vi "Traverse_to_Traverse_Collision.vi"(5 "Current Position":sgl[](array[numeric])=[0.0, 100.0, 40.0] format="%.2f", 7 "Traverse Name":string, 8 "Model  Roll        Pitch       Yaw (deg)":sgl[](array[numeric]) format="%#.2f", 9 "Work in Tunnel Coordinates":T1, 10 "Simulate/Run":T2=enum."Run VI", 11 "New Position":sgl[](array[numeric])=[0.0, 100.0, 40.0] format="%.2f") -> (1 "Error String":string)   [LabVIEW 2015]
uses:
  Controls/User_Specific_mode.ctl
  Controls/Tunnel_Coordinates.ctl
  Route mapping/Exclude_cluster.ctl
  Route mapping/Box_size.ctl
  Route mapping/Exclusion_type.ctl
  ADAM Client/Sub VIs/ADAM Controls/Quick_local_ADAM_Table.ctl
  Route mapping/Pict_Plot_Axis.ctl
  Route mapping/Axis.ctl
  Globals/Preference_global.vi
  Globals/Trav_pos_global.vi
panel:
  out "Plan View":picture
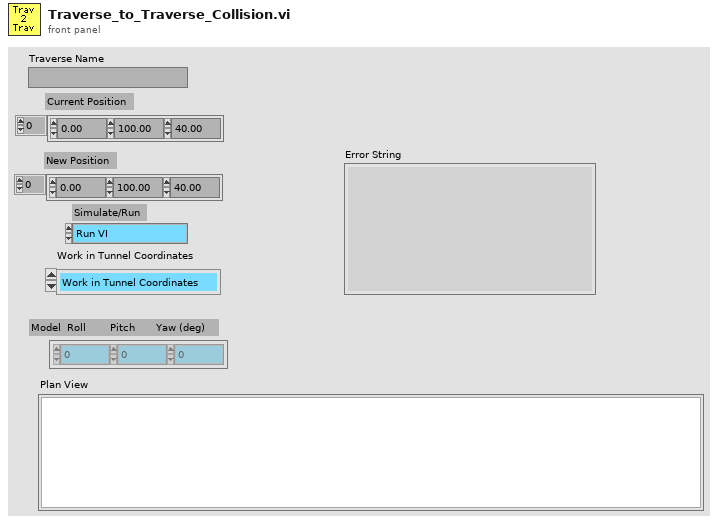
[diagram p1: front panel]
types:
  T1 = typedef "Tunnel_Coordinates.ctl" = enum16{"Work in Tunnel Coordinates", "Work in Model Coordinates"}
  T2 = typedef "User_Specific_mode.ctl" = enum16{"Check VI only", "Run VI"}
  T3 = typedef "Exclude_cluster.ctl" = cluster{"Sizes":T4, "Name":string, "Exclude Type":T5}
  T4 = typedef "Box_size.ctl" = cluster{"Max":sgl, "Min":sgl}[]
  T5 = typedef "Exclusion_type.ctl" = enum16{"Exclude completely", "Allow only vertical moves"}
  T6 = typedef "Quick_local_ADAM_Table.ctl" = enum16{"Read Global", "Load Global From ADAM Table", "Write Global"}
  T7 = enum16{"Load setup from excel file", "Save setup to excel file"}
  T8 = typedef "Pict_Plot_Axis.ctl" = cluster{"Width":T9, "Height":T9}
  T9 = typedef "Axis.ctl" = enum16{"X Axis", "X Axis -ve", "Y Axis", "Y Axis -ve", "Z Axis", "Z Axis -ve"}
  T10 = enum16{"To Traverse Coordinates", "To User Coordinates"}
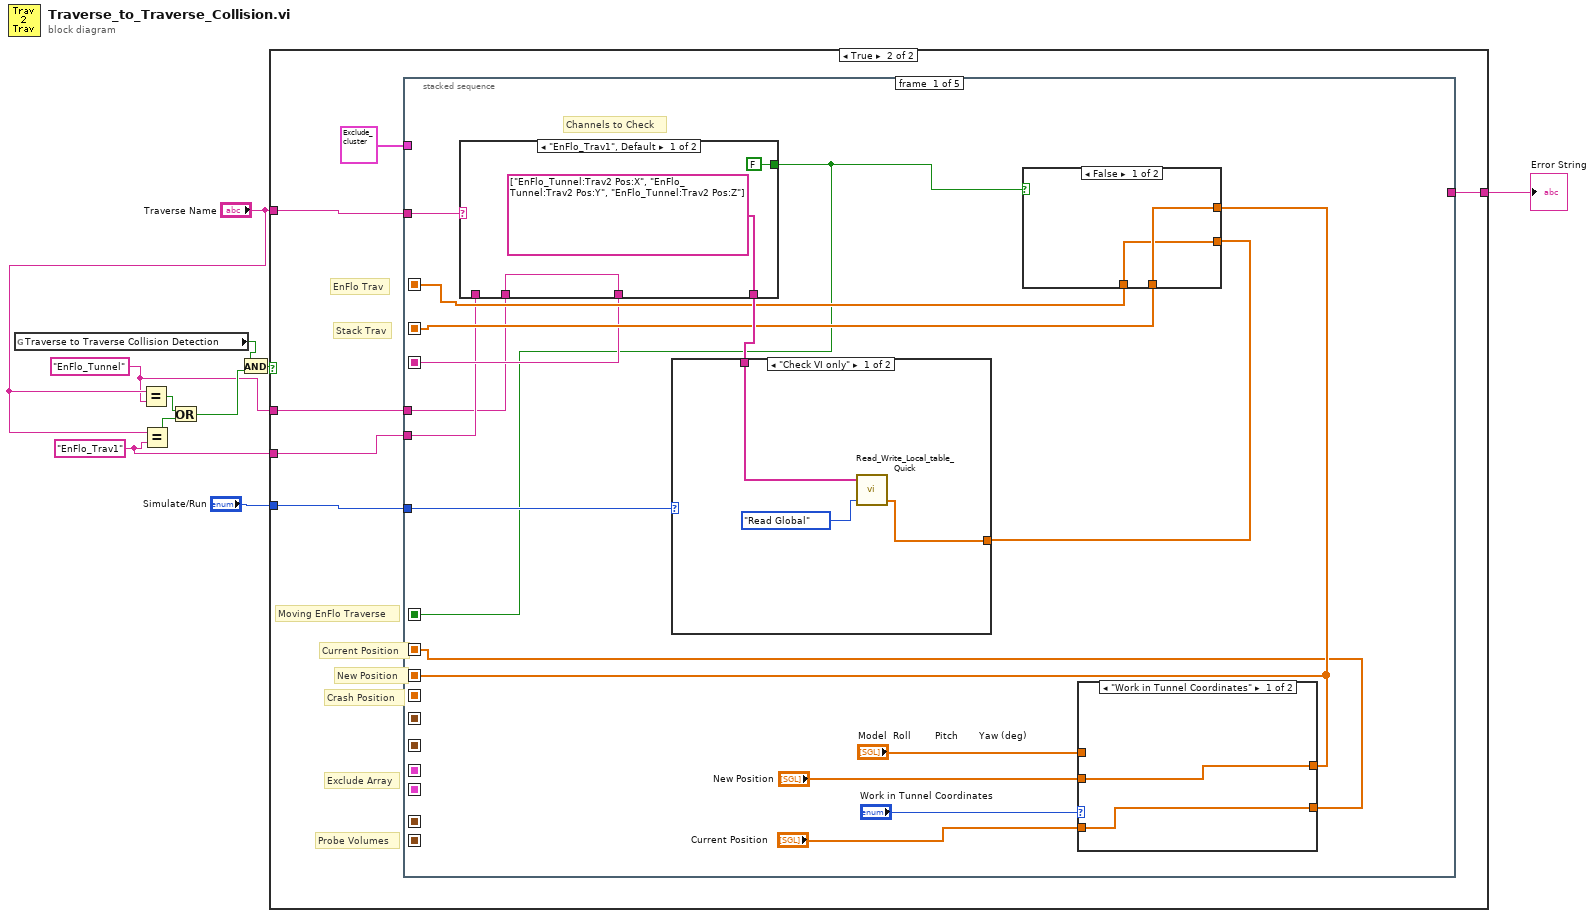
[diagram p0: block diagram]
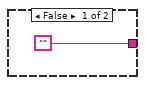
[diagram p2: hidden frame]
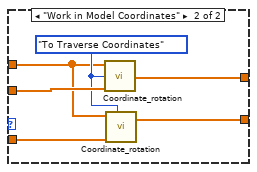
[diagram p4: hidden frame]
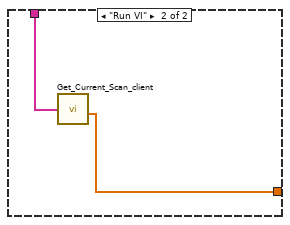
[diagram p5: hidden frame]
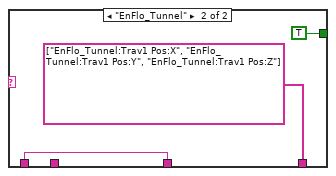
[diagram p6: hidden frame]
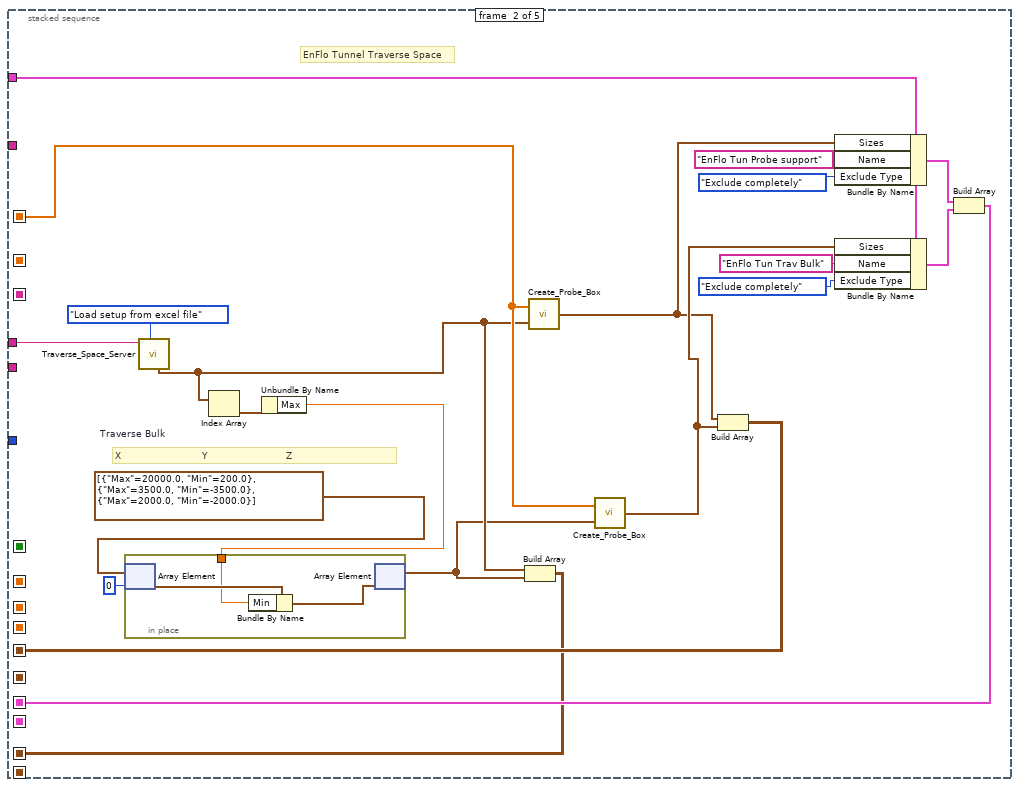
[diagram p7: hidden frame]
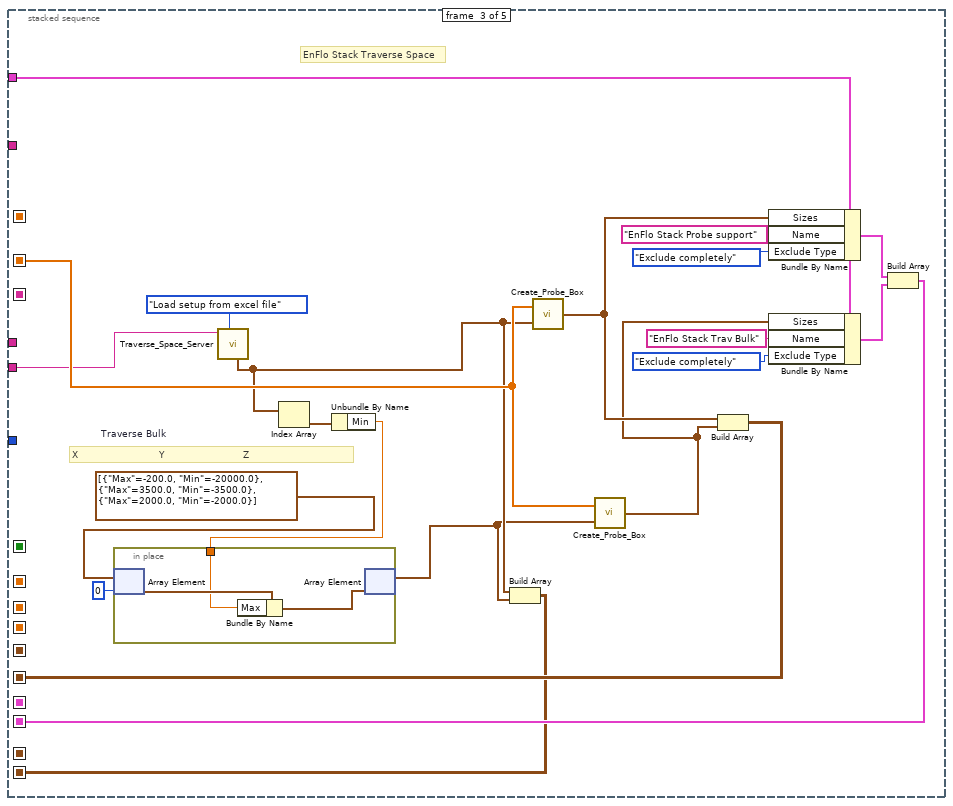
[diagram p8: hidden frame]
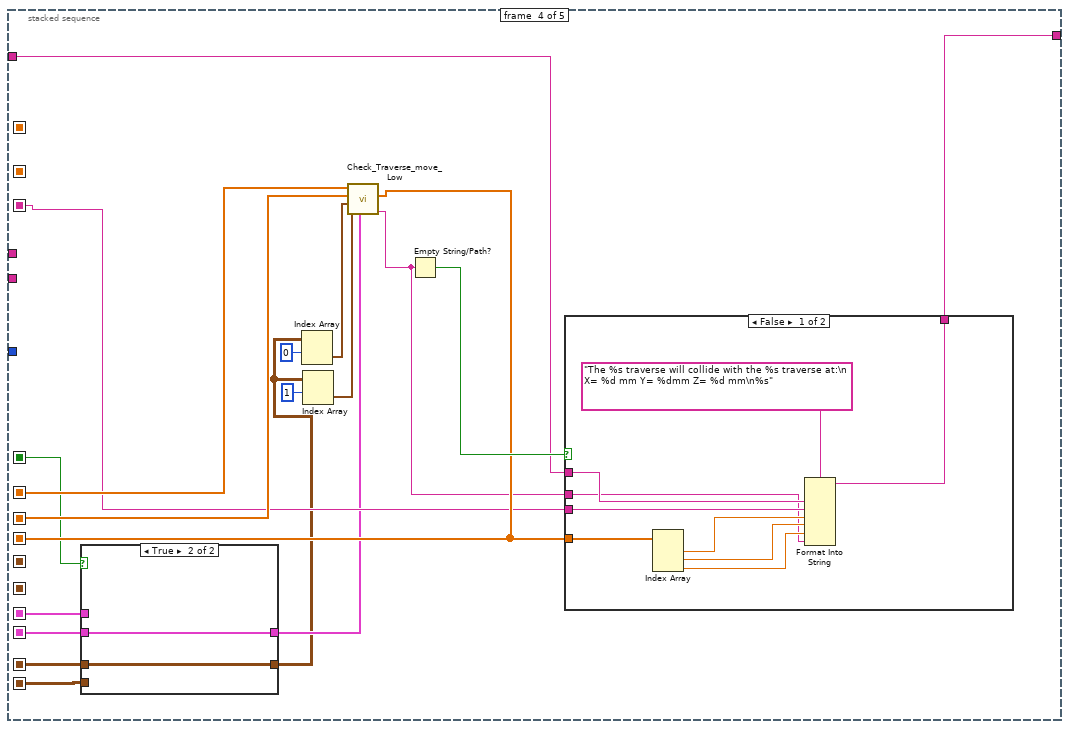
[diagram p9: hidden frame]
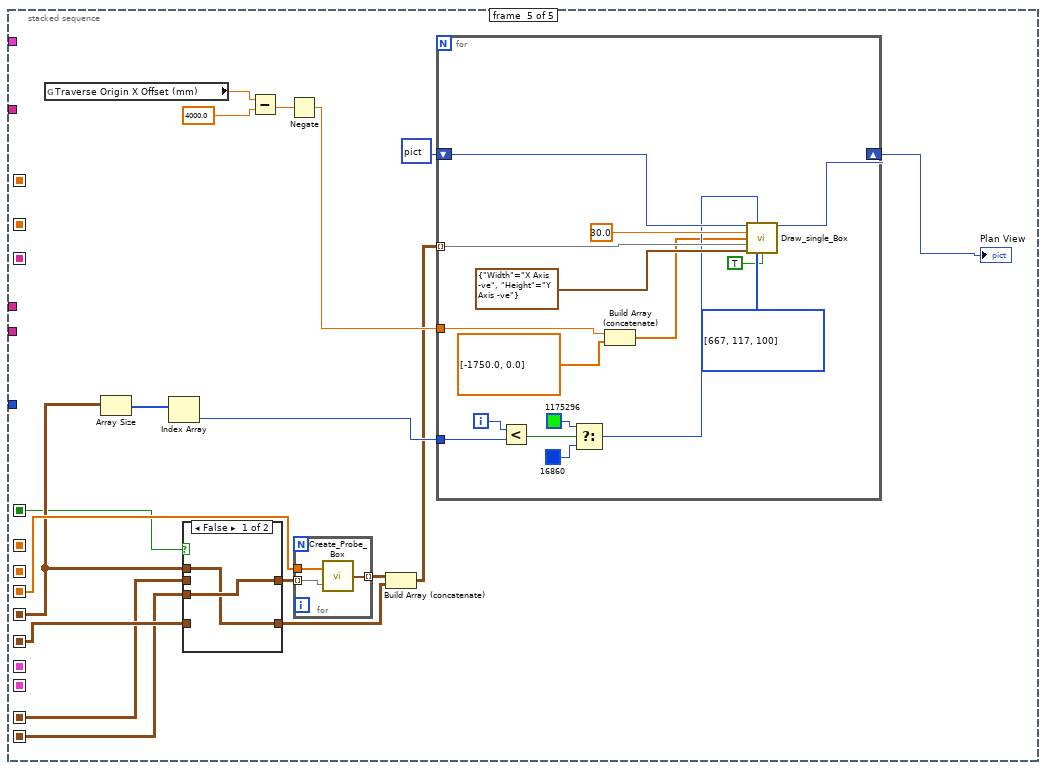
[diagram p12: hidden frame]
diagram:
  w2 = "EnFlo_Trav1" ("Rig Setup")
  w1 = "EnFlo_Tunnel" ("Rig Setup")
  n1 = global read "Preference_global.vi" "Traverse to Traverse Collision Detection"() -> (w7:bool)
  n2 = Equal?(x="Traverse Name", y=w1) -> (x = y?=w5:bool)
  n3 = Equal?(x="Traverse Name", y=w2) -> (x = y?=w4:bool)
  n4 = Or(x=w5, y=w4) -> (x .or. y?=w3:bool)
  n5 = And(x=w7, y=w3) -> (x .and. y?=w8:bool)
  n6 = case shown="True" w8 {
    tunnel: "Traverse Name" -> [_ w17]
    tunnel: "Simulate/Run" -> [_ w16]
    tunnel: ["" w15] -> w9
    tunnel: w2 -> [_ w13]
    tunnel: w1 -> [_ w12]
    frame False {
    }
    frame True {
      # "Moving EnFlo Traverse"
      # "Exclude Array"
      # "Probe Volumes"
      # "Crash Position"
      # "Current Position"
      # "New Position"
      # "Stack Trav"
      # "EnFlo Trav"
      n7 = stacked-sequence {
        seq-local: [w27 _ _ _ _] -> [_ w77 _ _ _]
        seq-local: [w26 _ _ _ _] -> [_ _ w100 _ _]
        seq-local: [_ w76 _ _ _] -> [_ _ _ _ w139]
        seq-local: [_ _ w101 _ _] -> [_ _ _ _ w146]
        seq-local: [w24 _ _ _ _] -> [_ _ _ w118 _]
        seq-local: [w23 _ _ _ _] -> [_ _ _ w123 _]
        seq-local: [_ _ w91 _ _] -> [_ _ _ w115 _]
        seq-local: [_ w66 _ _ _] -> [_ _ _ w113 _]
        seq-local: [_ w65 _ _ _] -> [_ _ _ w114 w144]
        seq-local: [_ _ w89 _ _] -> [_ _ _ w112 w140]
        seq-local: [w21 _ _ _ _] -> [_ _ _ w122 _]
        seq-local: [_ _ _ w120 _] -> [_ _ _ _ w141]
        seq-local: [w20 _ _ _ _] -> [_ _ _ w110 w138]
        tunnel: w17 -> [w31 _ _ w119 _]
        tunnel: w16 -> [w33 _ _ _ _]
        tunnel: [_ _ _ w117 _] -> w15
        tunnel: T3 {"Sizes"=[{"Max"=15000.0, "Min"=0.0}, {"Max"=1000.0, "Min"=-1000.0}, {"Max"=300.0, "Min"=0.0}], "Name"="Roughness Elements", "Exclude Type"=enum."Allow only vertical moves"} ("Cluster") -> [_ w67 w90 _ _]
        tunnel: w12 -> [w18 w64 _ _ _]
        tunnel: w13 -> [w19 _ w87 _ _]
        frame #0 {
          # "Channels to Check"
          n8 = case shown="\"EnFlo_Trav1\", Default" w31 {
            tunnel: [string[] ["EnFlo_Tunnel:Trav2 Pos:X", "EnFlo_Tunnel:Trav2 Pos:Y", "EnFlo_Tunnel:Trav2 Pos:Z"] string[] ["EnFlo_Tunnel:Trav1 Pos:X", "EnFlo_Tunnel:Trav1 Pos:Y", "EnFlo_Tunnel:Trav1 Pos:Z"]] -> w32
            tunnel: [FALSE TRUE] -> w20
            tunnel: [w51 w54] -> w24
            tunnel: w19 -> [_ w54]
            tunnel: w18 -> [w51 _]
            frame "EnFlo_Trav1", Default {
            }
            frame "EnFlo_Tunnel" {
            }
          }
          n9 = case shown="\"Check VI only\"" w33 {
            tunnel: [w46 w49] -> w25
            tunnel: w32 -> [w47 w50]
            frame "Check VI only" {
              n10 = call "Read_Write_Local_table_Quick.vi"("Mode"=Quick_local_ADAM_Table."Read Global", "Ch names In"=w47) -> ("Numeric Values Out"=w46:dbl[])  [unwired: 1 in, 2 out]
            }
            frame "Run VI" {
              n11 = call "Get_Current_Scan_client.vi"("ADAM Ch Names"=w50) -> ("Numerical Values"=w49:dbl[])  [unwired: 3 out]
            }
          }
          n12 = case shown="\"Work in Tunnel Coordinates\"" "Work in Tunnel Coordinates" {
            tunnel: "Model  Roll        Pitch       Yaw (deg)" -> [_ w42]
            tunnel: "New Position" -> [w39 w45]
            tunnel: [w39 w44] -> w23
            tunnel: "Current Position" -> [w38 w41]
            tunnel: [w38 w40] -> w21
            frame "Work in Tunnel Coordinates" {
            }
            frame "Work in Model Coordinates" {
              w43 = T10."To Traverse Coordinates" ("Mode")
              n13 = call "Coordinate_rotation.vi"("Roll-Pitch-Yaw"=w42, "Input Position"=w45, "Mode"=w43) -> ("Output Position"=w44:sgl[])  [unwired: 2 in, 1 out]
              n14 = call "Coordinate_rotation.vi"("Roll-Pitch-Yaw"=w42, "Input Position"=w41, "Mode"=w43) -> ("Output Position"=w40:sgl[])  [unwired: 2 in, 1 out]
            }
          }
          n15 = case shown="False" w20 {
            tunnel: [w34 w37] -> w27
            tunnel: w23 -> [w35 w37]
            tunnel: [w35 w36] -> w26
            tunnel: w25 -> [w34 w36]
            frame False {
            }
            frame True {
            }
          }
        }
        frame #1 {
          w60 = T4 [{"Max"=20000.0, "Min"=200.0}, {"Max"=3500.0, "Min"=-3500.0}, {"Max"=2000.0, "Min"=-2000.0}]  # Traverse Bulk
          # "X                           Y                          Z"
          # "EnFlo Tunnel Traverse Space"
          n16 = call "Traverse_Space_Server.vi"("Mode"=T7."Load setup from excel file", "Traverse Name"=w64) -> ("Probe Support Out"=w62:T4)  [unwired: 4 in, 5 out]
          n17 = Index Array(array=w62) -> (element=w61:cluster{"Max":sgl, "Min":sgl})  [unwired: 1 in]
          n18 = Unbundle By Name(w61) -> ("Max"=w57:sgl)
          n19 = in-place {
            in-place-border: w57 -> [w79]
            n20 = in-place-array #1(w60, 0) -> (w80:cluster{"Max":sgl, "Min":sgl})
            n21 = Bundle By Name(cluster=w80, "Min"=w79) -> (w78:cluster{"Max":sgl, "Min":sgl})
            n22 = in-place-array #1(w78) -> (w59:T4)  [unwired: 1 out]
          }
          n23 = Build Array(w62, w59) -> (w65:cluster{"Max":sgl, "Min":sgl}[][])
          n24 = call "Create_Probe_Box.vi"("Probe Volume"=w62, "Probe Position"=w77) -> ("Current Probe Volume"=w68:T4)
          n25 = call "Create_Probe_Box.vi"("Probe Volume"=w59, "Probe Position"=w77) -> ("Current Probe Volume"=w69:T4)
          n26 = Build Array(w68, w69) -> (w76:cluster{"Max":sgl, "Min":sgl}[][])
          n27 = Bundle By Name(cluster=w67, "Sizes"=w68, "Name"="EnFlo Tun Probe support", "Exclude Type"=Exclusion_type."Exclude completely") -> (w70:T3)
          n28 = Bundle By Name(cluster=w67, "Sizes"=w69, "Name"="EnFlo Tun Trav Bulk", "Exclude Type"=Exclusion_type."Exclude completely") -> (w71:T3)
          n29 = Build Array(w70, w71) -> (w66:T3[])
        }
        frame #2 {
          w84 = T4 [{"Max"=-200.0, "Min"=-20000.0}, {"Max"=3500.0, "Min"=-3500.0}, {"Max"=2000.0, "Min"=-2000.0}]  # Traverse Bulk
          # "X                           Y                          Z"
          # "EnFlo Stack Traverse Space"
          n30 = call "Traverse_Space_Server.vi"("Mode"=T7."Load setup from excel file", "Traverse Name"=w87) -> ("Probe Support Out"=w85:T4)  [unwired: 4 in, 5 out]
          n31 = Index Array(array=w85) -> (element=w86:cluster{"Max":sgl, "Min":sgl})  [unwired: 1 in]
          n32 = Unbundle By Name(w86) -> ("Min"=w82:sgl)
          n33 = in-place {
            in-place-border: w82 -> [w103]
            n34 = in-place-array #2(w84, 0) -> (w104:cluster{"Max":sgl, "Min":sgl})
            n35 = Bundle By Name(cluster=w104, "Max"=w103) -> (w102:cluster{"Max":sgl, "Min":sgl})
            n36 = in-place-array #2(w102) -> (w81:T4)  [unwired: 1 out]
          }
          n37 = Build Array(w85, w81) -> (w89:cluster{"Max":sgl, "Min":sgl}[][])
          n38 = call "Create_Probe_Box.vi"("Probe Volume"=w85, "Probe Position"=w100) -> ("Current Probe Volume"=w99:T4)
          n39 = call "Create_Probe_Box.vi"("Probe Volume"=w81, "Probe Position"=w100) -> ("Current Probe Volume"=w95:T4)
          n40 = Build Array(w99, w95) -> (w101:cluster{"Max":sgl, "Min":sgl}[][])
          n41 = Bundle By Name(cluster=w90, "Sizes"=w99, "Name"="EnFlo Stack Probe support", "Exclude Type"=Exclusion_type."Exclude completely") -> (w92:T3)
          n42 = Bundle By Name(cluster=w90, "Sizes"=w95, "Name"="EnFlo Stack Trav Bulk", "Exclude Type"=Exclusion_type."Exclude completely") -> (w93:T3)
          n43 = Build Array(w92, w93) -> (w91:T3[])
        }
        frame #3 {
          n44 = case shown="True" w110 {
            tunnel: [w125 w127] -> w116
            tunnel: w115 -> [_ w127]
            tunnel: [w124 w126] -> w105
            tunnel: w114 -> [_ w126]
            tunnel: w113 -> [w125 _]
            tunnel: w112 -> [w124 _]
            frame False {
            }
            frame True {
            }
          }
          n45 = Index Array(array=w105, index (row)=0) -> (element=w107:cluster{"Max":sgl, "Min":sgl}[])  [unwired: 1 in]
          n46 = Index Array(array=w105, index (row)=1) -> (element=w106:cluster{"Max":sgl, "Min":sgl}[])  [unwired: 1 in]
          n47 = call "Check_Traverse_move_Low.vi"("Exclude Array"=w116, "Probe Support"=w106, "Probe Volume"=w107, "New Position"=w123, "Current position"=w122) -> ("Error Comments"=w111:string, "Position At Crash"=w120:dbl[])  [unwired: 3 in]
          n48 = Empty String/Path?(string/path=w111) -> (empty?=w121:bool)
          n49 = case shown="False" w121 {
            tunnel: [w134 w137] -> w117
            tunnel: w111 -> [w128 w137]
            tunnel: w119 -> [w129 _]
            tunnel: w118 -> [w135 _]
            tunnel: w120 -> [w133 _]
            frame False {
              n50 = Index Array(array=w133) -> (element #1=w130:dbl, element #2=w132:dbl, element #3=w131:dbl)  [unwired: 3 in]
              n51 = Format Into String(format string="The %s traverse will collide with the %s traverse at:\n X= %d mm Y= %dmm Z= %d mm\n%s" ("Format String"), w129, w135, w130, w132, w131, w128) -> (resulting string=w134:string)  [unwired: 2 in, 1 out]
            }
            frame True {
            }
          }
        }
        frame #4 {
          n52 = global read "Trav_pos_global.vi" "Traverse Origin X Offset (mm)"() -> (w150:sgl)
          n53 = Array Size(array=w139) -> (size(s)=w153:i32[])
          n54 = Index Array(array=w153) -> (element=w152:i32)  [unwired: 1 in]
          n55 = case shown="False" w138 {
            tunnel: [w159 w162] -> w147
            tunnel: w146 -> [_ w162]
            tunnel: w144 -> [_ w161]
            tunnel: [w160 w161] -> w143
            tunnel: w140 -> [w160 _]
            tunnel: w139 -> [w159 _]
            frame False {
            }
            frame True {
            }
          }
          n56 = Subtract(x=w150, y=4000.0 ("x")) -> (x-y=w148:dbl)
          n57 = Negate(x=w148) -> (-x=w151:dbl)
          n58 = for {
            tunnel: w143 -> [w158] mode=indexing
            tunnel: [w157] -> w142 mode=indexing
            tunnel: w141 -> [w156]
            n59 = call "Create_Probe_Box.vi"("Probe Volume"=w158, "Probe Position"=w156) -> ("Current Probe Volume"=w157:T4)
          }
          n60 = Build Array (concatenate)(w142, w147) -> (w145:cluster{"Max":sgl, "Min":sgl}[][])
          n61 = for {
            shift-right: [w175] -> w154
            shift-left: picture data[5B] ("Picture in") -> [w176]
            tunnel: w145 -> [w174] mode=indexing
            tunnel: w152 -> [w170]
            tunnel: w151 -> [w164]
            i -> [w171]
            n62 = Less?(x=w171, y=w170) -> (x < y?=w169:bool)
            n63 = Select(t=u32 1175296 ("color(black)"), s=w169, f=u32 16860 ("color(black)")) -> (s? t:f=w166:u32)
            n64 = Build Array (concatenate)(w164, dbl[] [-1750.0, 0.0] ("Min Values")) -> (w163:dbl[])
            n65 = call "Draw_single_Box.vi"("Picture in"=w176, "color(black)"=w166, "mm Per Pixel"=30.0, "Min Values"=w163, "Box Coordinates"=w174, "View"=T8 {"Width"=enum."X Axis -ve", "Height"=enum."Y Axis -ve"}, "Pixels per Axis"=i16[] [667, 117, 100], "fill?(F)"=TRUE) -> ("Picture out"=w175:picture)  [unwired: 7 out]
          }
          "Plan View" <- w154
        }
      }
    }
  }
  "Error String" <- w9
